vi "Menu.Properties.Load.vi"(8 "error in (no error)":errorcluster, 9 "Menu in":refnum<k9>, 10 "Coords":T1, 11 "Cluster in":T2) -> (0 "error out":errorcluster, 3 "Cluster out":T2)   [LabVIEW 2013, in "Simple Sequence Editor.lvlib"]
uses:
  Simple Sequence Editor.lvlib
  Types/StateVariables.ctl
  Types/ChannelProperties.ctl
  <vilib>/Utility/miscctls.llb/LVPoint32TypeDef.ctl
  Constants.vi
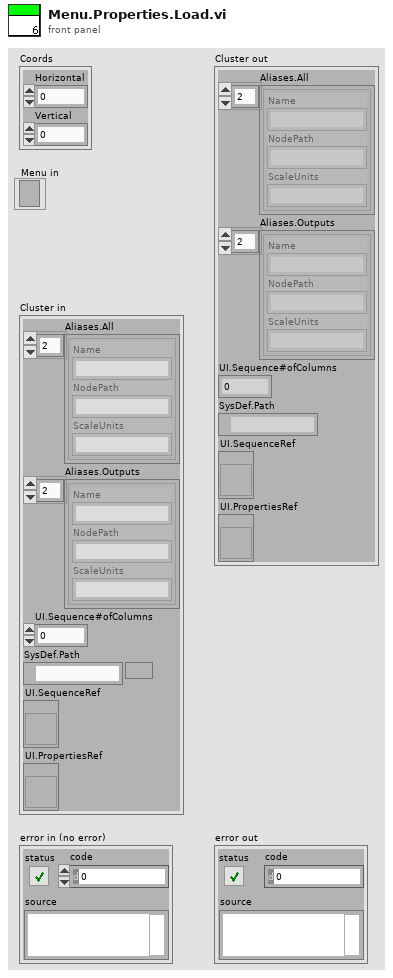
[diagram p1: front panel]
types:
  T1 = typedef "LVPoint32TypeDef.ctl" = cluster{"Horizontal":i32, "Vertical":i32}
  T2 = typedef "Simple Sequence Editor.lvlib/StateVariables.ctl" = cluster{"Aliases.All":T3[], "Aliases.Outputs":T3[], "UI.Sequence#ofColumns":i32, "SysDef.Path":path, "UI.SequenceRef":refnum<vi>, "UI.PropertiesRef":refnum<vi>}
  T3 = typedef "Simple Sequence Editor.lvlib/ChannelProperties.ctl" = cluster{"Name":string, "NodePath":string, "ScaleUnits":string}
  T4 = typedef "LVRowAndColumnTypeDef.ctl" = cluster{"Row":i32, "Column":i32}
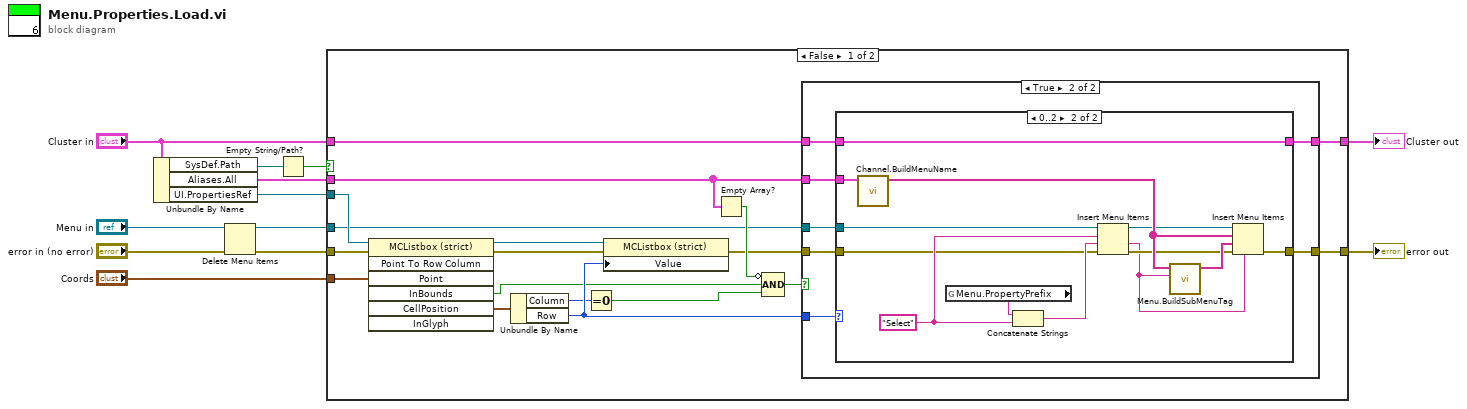
[diagram p0: block diagram]
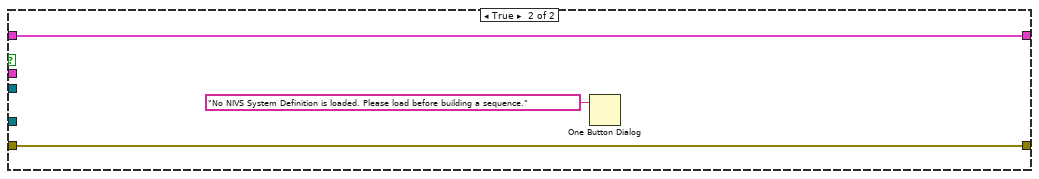
[diagram p4: hidden frame]
diagram:
  n1 = Unbundle By Name("Cluster in") -> ("SysDef.Path"=w12:path, "Aliases.All"=w11:T3[], "UI.PropertiesRef"=w6:refnum<vi>)
  n2 = Delete Menu Items(6:"error in (no error)", 9:"Menu in") -> (0:w1:errorcluster, 3:w2:refnum<k9>)  [unwired: 2 in]
  n3 = Empty String/Path?(string/path=w12) -> (empty?=w5:bool)
  n4 = case shown="False" w5 {
    tunnel: w11 -> [w16 _]
    tunnel: "Cluster in" -> [w30 w56]
    tunnel: [w26 w55] -> w9
    tunnel: w1 -> [w25 w55]
    tunnel: [w24 w56] -> w8
    tunnel: w2 -> [w13 _]
    tunnel: "Coords" -> [w18 _]
    tunnel: w6 -> [w17 _]
    frame False {
      n5 = invoke class="MCListbox (strict)" method="Point To Row Column"(reference=w17, error in=w25, "Point"=w18) -> (reference out=w27:refnum<vi>, error out=w29:errorcluster, "InBounds"=w20:bool, "CellPosition"=w19:T4)  [unwired: 4 in, 3 out]
      n6 = Unbundle By Name(w19) -> ("Column"=w21:i32, "Row"=w28:i32)
      n7 = Equal To 0?(x=w21) -> (x = 0?=w22:bool)
      n8 = property class="MCListbox (strict)"(reference=w27, error in=w29, "Value"=w28) -> (error out=w14:errorcluster)  [unwired: 1 out]
      n9 = Empty Array?(array=w16) -> (empty?=w15:bool)
      n10 = Compound Arithmetic op=AND(invert w15, w20, w22) -> (w23:bool)
      n11 = case shown="True" w23 {
        tunnel: w28 -> [_ w39]
        tunnel: w13 -> [_ w37]
        tunnel: w30 -> [w32 w38]
        tunnel: w14 -> [w31 w36]
        tunnel: [w32 w35] -> w24
        tunnel: [w31 w34] -> w26
        tunnel: w16 -> [_ w33]
        frame False {
        }
        frame True {
          n12 = case shown="0..2" w39 {
            tunnel: w38 -> [w41 w44]
            tunnel: w37 -> [_ w54]
            tunnel: w36 -> [w40 w46]
            tunnel: [w41 w44] -> w35
            tunnel: [w40 w43] -> w34
            tunnel: w33 -> [_ w42]
            frame Default {
            }
            frame 0..2 {
              w52 = "Select" ("string")
              n13 = call "Channel.BuildMenuName.vi"("Aliases"=w42) -> ("Aliases Array"=w49:string[])  [unwired: 10 in]
              n14 = global read "Constants.vi" "Menu.PropertyPrefix"() -> (w53:string)
              n15 = Concatenate Strings(w53, w52) -> (w51:string)
              n16 = Insert Menu Items(6:w46, 7:w51, 8:w52, 9:w54) -> (0:w47:errorcluster, 1:w45:string, 3:w48:refnum<k9>)  [unwired: 2 in]
              n17 = call "Menu.BuildSubMenuTag.vi"("Menu"=w45, "Aliases Array"=w49) -> ("Tag Array"=w50:string[])  [unwired: 9 in]
              n18 = Insert Menu Items(5:w45, 6:w47, 7:w50, 8:w49, 9:w48) -> (0:w43:errorcluster)  [unwired: 1 in, 2 out]
            }
          }
        }
      }
    }
    frame True {
      n19 = One Button Dialog(message="No NIVS System Definition is loaded. Please load before building a sequence.") -> ()  [unwired: 1 in, 1 out]
    }
  }
  "error out" <- w9
  "Cluster out" <- w8
